vi "accurus_control_vacuum.vi"(7 "Irrigate?":bool=TRUE, 8 "Max Limit [mmHg]":dbl, 9 "stop":bool=TRUE, 10 "vacuum force":i8, 11 "Slide in":refnum<vi>) -> (1 "f":dbl, 2 "f 2":dbl, 3 "f 3":dbl, 4 "Boolean":bool, 5 "Boolean 2":bool, 6 "Vacuum Force\n[mmHg]":i32)   [LabVIEW 2016]
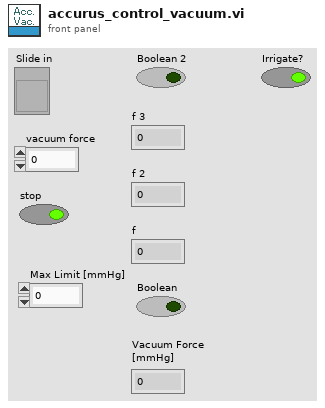
[diagram p1: front panel]
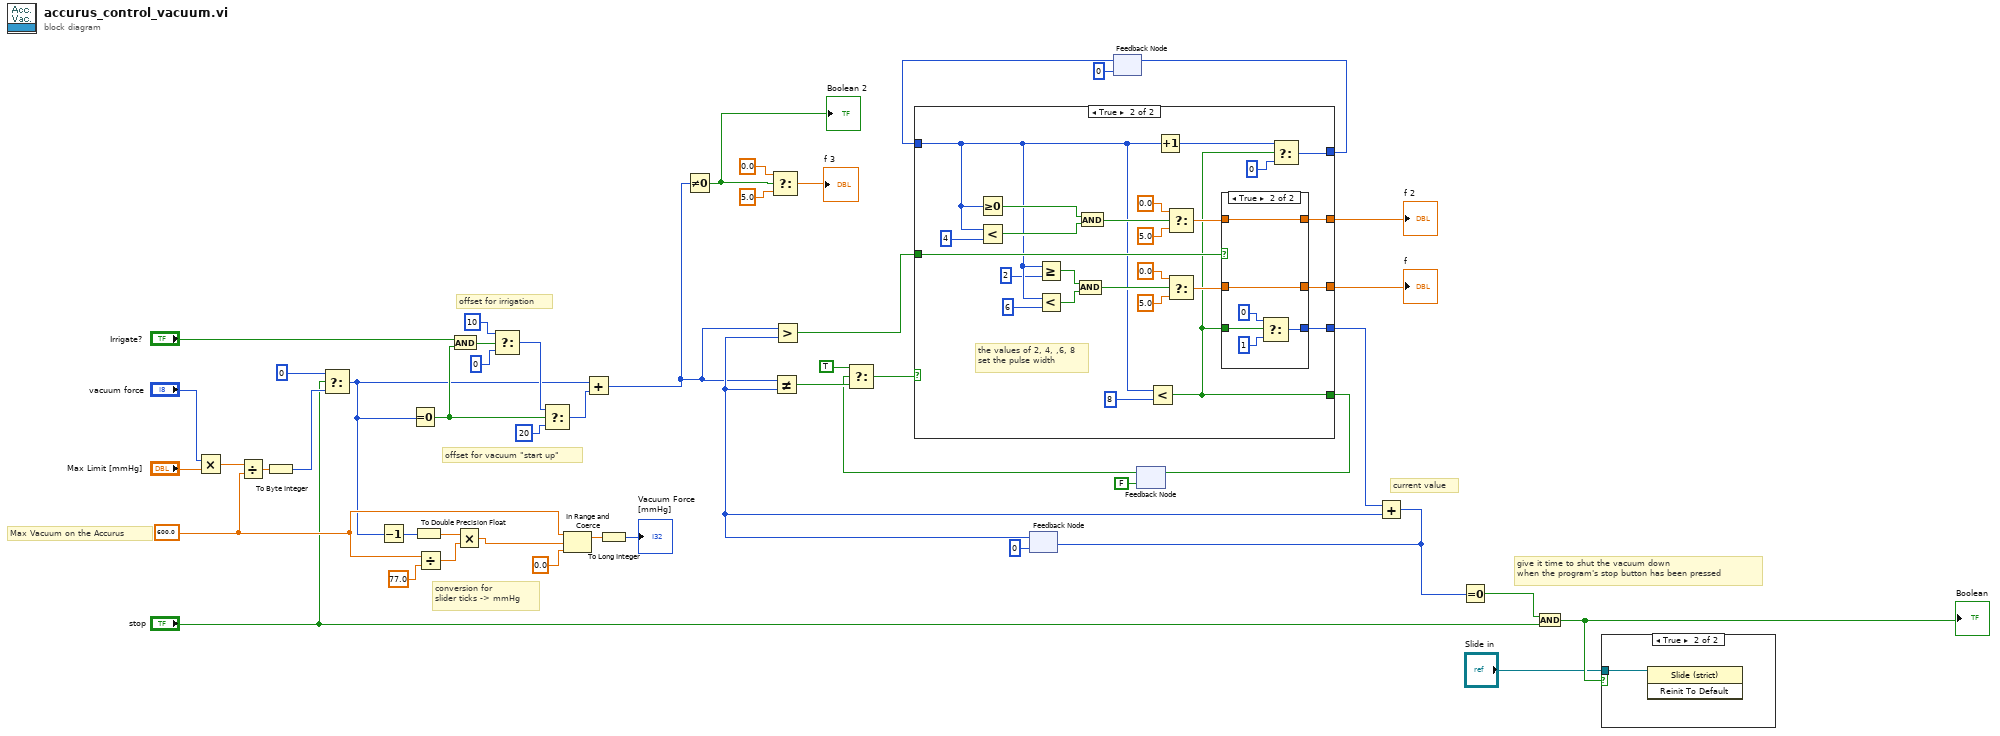
[diagram p0: block diagram]
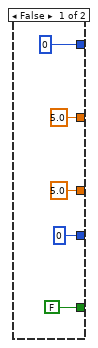
[diagram p3: hidden frame]
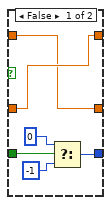
[diagram p4: hidden frame]
diagram:
  w14 = 600.0
  # "offset for irrigation"
  # "Max Vacuum on the Accurus"
  # "give it time to shut the vacuum down \nwhen the program's stop button has been pressed"
  # "conversion for\nslider ticks -> mmHg"
  # "offset for vacuum \"start up\""
  # "current value"
  n1 = Multiply(x="vacuum force", y="Max Limit [mmHg]") -> (x*y=w15:dbl)
  n2 = Divide(x=w15, y=w14) -> (x/y=w13:dbl)
  n3 = To Byte Integer(number=w13) -> (8bit integer=w4:i8)
  n4 = Select(t=i8 0, s="stop", f=w4) -> (s? t:f=w3:i8)
  n5 = Decrement(x=w3) -> (x-1=w20:i8)
  n6 = Equal To 0?(x=w3) -> (x = 0?=w11:bool)
  n7 = To Double Precision Float(number=w20) -> (double precision float=w49:dbl)
  n8 = Divide(x=w14, y=77.0) -> (x/y=w18:dbl)
  n9 = And(x="Irrigate?", y=w11) -> (x .and. y?=w10:bool)
  n10 = Multiply(x=w49, y=w18) -> (x*y=w17:dbl)
  n11 = Select(t=i8 10, s=w10, f=i8 0 ("t")) -> (s? t:f=w6:i8)
  n12 = Select(t=w6, s=w11, f=i8 20) -> (s? t:f=w44:i8)
  n13 = In Range and Coerce(upper limit=w14, x=w17, lower limit=0.0) -> (coerced(x)=w21:dbl)  [unwired: 1 out]
  n14 = Add(x=w3, y=w44) -> (x+y=w5:i8)
  n15 = To Long Integer(number=w21) -> (32bit integer=→"Vacuum Force\n[mmHg]":i32)
  n16 = Not Equal To 0?(x=w5) -> (x != 0?=w7:bool)
  "Boolean 2" <- w7
  n17 = Select(t=0.0, s=w7, f=5.0) -> (s? t:f=→"f 3":dbl)
  n18 = feedback #1(i8 0) -> (w30:i8)
  n19 = Not Equal?(x=w5, y=w30) -> (x != y?=w36:bool)
  n20 = Greater?(x=w5, y=w30) -> (0:w26:bool)
  n21 = feedback #2(i8 0) -> (w32:i8)
  n22 = feedback #3(FALSE) -> (w33:bool)
  n23 = Select(t=TRUE, s=w33, f=w36) -> (s? t:f=w35:bool)
  n24 = case shown="True" w35 {
    tunnel: [5.0 ("f") w67] -> w40
    tunnel: [5.0 ("f") w66] -> w41
    tunnel: [i8 0 ("f") w64] -> w29
    tunnel: [FALSE w59] -> w25
    tunnel: w26 -> [_ w65]
    tunnel: [i8 0 w61] -> w27
    tunnel: w32 -> [_ w63]
    frame False {
    }
    frame True {
      # "the values of 2, 4, ,6, 8 \nset the pulse width"
      n25 = Greater Or Equal To 0?(x=w63) -> (x >= 0?=w74:bool)
      n26 = Less?(x=w63, y=i8 4) -> (x < y?=w73:bool)
      n27 = Greater Or Equal?(x=w63, y=i8 2) -> (x >= y?=w72:bool)
      n28 = Less?(x=w63, y=i8 6) -> (x < y?=w71:bool)
      n29 = And(x=w72, y=w71) -> (x .and. y?=w70:bool)
      n30 = And(x=w74, y=w73) -> (x .and. y?=w75:bool)
      n31 = Less?(x=w63, y=i8 8) -> (x < y?=w59:bool)
      n32 = Increment(x=w63) -> (x+1=w62:i8)
      n33 = Select(t=0.0, s=w75, f=5.0) -> (s? t:f=w69:dbl)
      n34 = Select(t=0.0, s=w70, f=5.0) -> (s? t:f=w68:dbl)
      n35 = case shown="True" w65 {
        tunnel: w69 -> [w84 w90]
        tunnel: w68 -> [w85 w91]
        tunnel: [w84 w91] -> w66
        tunnel: [w85 w90] -> w67
        tunnel: w59 -> [w80 w89]
        tunnel: [w81 w88] -> w64
        frame False {
          n36 = Select(t=i8 0, s=w80, f=i8 -1) -> (s? t:f=w81:i8)
        }
        frame True {
          n37 = Select(t=i8 0, s=w89, f=i8 1) -> (s? t:f=w88:i8)
        }
      }
      n38 = Select(t=w62, s=w59, f=i8 0) -> (s? t:f=w61:i8)
    }
  }
  "f" <- w41
  "f 2" <- w40
  n39 = feedback-in #2(w27) -> ()
  n40 = feedback-in #3(w25) -> ()
  n41 = Add(x=w29, y=w30) -> (x+y=w46:i8)
  n42 = feedback-in #1(w46) -> ()
  n43 = Equal To 0?(x=w46) -> (x = 0?=w47:bool)
  n44 = And(x=w47, y="stop") -> (x .and. y?=w48:bool)
  "Boolean" <- w48
  n45 = case shown="True" w48 {
    tunnel: "Slide in" -> [_ w92]
    frame False {
    }
    frame True {
      n46 = invoke on="Invoke Node" class="Slide (strict)" method="Reinit To Default"(reference=w92) -> ()  [unwired: 2 in, 3 out]
    }
  }
